vi "Ingestion Config.vi"(10 "Data":string) -> (2 "Message":string)   [LabVIEW 2024, in "Sift Client.lvlib"]
uses:
  Sift Client.lvlib
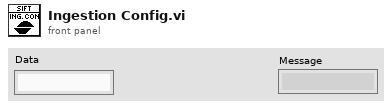
[diagram p1: front panel]
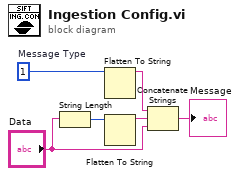
[diagram p0: block diagram]
diagram:
  w5 = u8 1  # Message Type
  n1 = String Length(string="Data") -> (length=w6:i32)
  n2 = Flatten To String(anything=w5) -> (data string=w4:string)  [unwired: 3 in, 2 out]
  n3 = Flatten To String(anything=w6) -> (data string=w3:string)  [unwired: 3 in, 2 out]
  n4 = Concatenate Strings(w4, w3, "Data") -> (→"Message":string)
